vi "Drop.vi"() -> ()   [LabVIEW 2013]
uses:
  Robot Global Data.vi
panel:
  in  "Close Charles Angle (Degrees)":dbl=130.0
  in  "Close Charles Time":u32=500
  in  "Lift Arm Time":u32=300
  in  "Open Charles Time":u32=200
  out "Start Time":u32
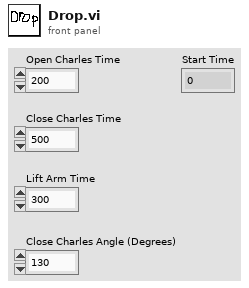
[diagram p1: front panel]
types:
  T1 = cluster{"Axes":cluster{"LS X":dbl, "LS Y":dbl, "Triggers":dbl, "RS X":dbl, "RS Y":dbl}, "Buttons":cluster{"LT":bool, "RT":bool, "A":bool, "B":bool, "X":bool, "Y":bool, "LB":bool, "RB":bool, "Back":bool, "Start":bool, "LS":bool, "RS":bool}, "Buttons Just Pushed":cluster{"LT":bool, "RT":bool, "A":bool, "B":bool, "X":bool, "Y":bool, "LB":bool, "RB":bool, "Back":bool, "Start":bool, "LS":bool, "RS":bool}}
  T2 = enum16{"Hold", "Pick Up", "Catch", "Aim", "Shoot"}
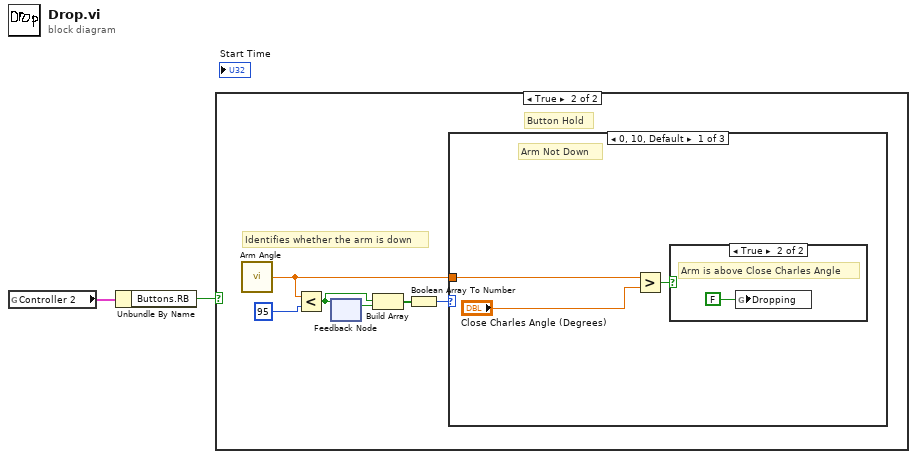
[diagram p0: block diagram]
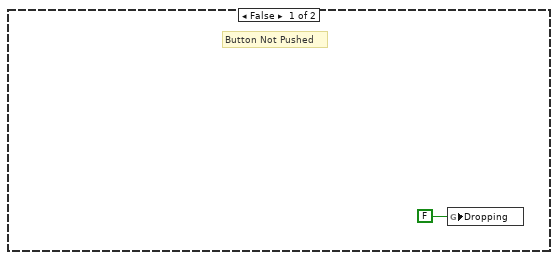
[diagram p2: hidden frame]
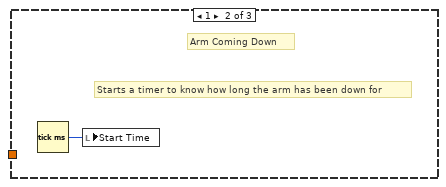
[diagram p4: hidden frame]
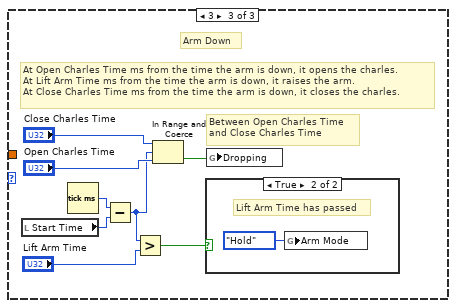
[diagram p5: hidden frame]
diagram:
  n1 = global read "Robot Global Data.vi" "Controller 2"() -> (w2:T1)
  n2 = Unbundle By Name(w2) -> ("Buttons.RB"=w1:bool)
  n3 = case shown="True" w1 {
    frame False {
      # "Button Not Pushed"
      n4 = global write "Robot Global Data.vi" "Dropping"(FALSE) -> ()
    }
    frame True {
      # "Button Hold"
      # "Identifies whether the arm is down"
      n5 = call "Arm Angle.vi"() -> ("Angle"=w5:dbl)  [unwired: 1 in, 2 out]
      n6 = Less?(x=w5, y=95) -> (x < y?=w6:bool)
      n7 = feedback #1() -> (w8:bool)  [unwired: 1 in]
      n8 = feedback-in #1(w6) -> ()
      n9 = Build Array(w6, w8) -> (w9:bool[])
      n10 = Boolean Array To Number(Boolean array=w9) -> (number=w7:u32)
      n11 = case shown="0, 10, Default" w7 {
        tunnel: w5 -> [w12 _ _]
        frame 0, 2, Default {
          # "Arm Not Down"
          n12 = Greater?(x=w12, y="Close Charles Angle (Degrees)") -> (0:w11:bool)
          n13 = case shown="True" w11 {
            frame False {
              # "Arm is below Close Charles Angle"
            }
            frame True {
              # "Arm is above Close Charles Angle"
              n14 = global write "Robot Global Data.vi" "Dropping"(FALSE) -> ()
            }
          }
        }
        frame 1 {
          # "Arm Coming Down"
          # "Starts a timer to know how long the arm has been down for"
          n15 = Tick Count (ms)() -> (millisecond timer value=w14:u32)
          n16 = local write "Start Time"(w14) -> ()
        }
        frame 3 {
          # "Between Open Charles Time\nand Close Charles Time"
          # "Arm Down"
          # "At Open Charles Time ms from the time the arm is down, it opens the charles.\nAt Lift Arm Time ms from the time the arm is down, it raises the arm.\nAt Close Charles Time ms from the time the arm is down, it closes the charles."
          n17 = local read "Start Time"() -> (w22:u32)
          n18 = Tick Count (ms)() -> (millisecond timer value=w21:u32)
          n19 = Subtract(x=w21, y=w22) -> (x-y=w16:u32)
          n20 = Greater?(x=w16, y="Lift Arm Time") -> (0:w19:bool)
          n21 = In Range and Coerce(upper limit="Close Charles Time", x=w16, lower limit="Open Charles Time") -> (In Range?=w15:bool)  [unwired: 1 out]
          n22 = case shown="True" w19 {
            frame False {
              # "Lift Arm Time hasn't passed"
            }
            frame True {
              # "Lift Arm Time has passed"
              n23 = global write "Robot Global Data.vi" "Arm Mode"(T2."Hold" ("Arm Mode")) -> ()
            }
          }
          n24 = global write "Robot Global Data.vi" "Dropping"(w15) -> ()
        }
      }
    }
  }
